vi "Path to String.vi"(1 "Path":path) -> (0 "Path String":string)   [LabVIEW 2020, in "feature_detection.lvlib" / "WeChat QR Code Detector.lvclass"]
uses:
  WeChat QR Code Detector.lvclass
  WeChat QR Code Detector.lvclass/WeChat QR Code Detector.ctl
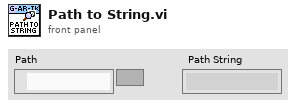
[diagram p1: front panel]
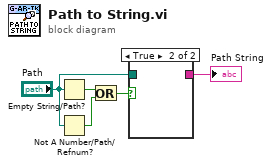
[diagram p0: block diagram]
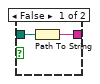
[diagram p2: hidden frame]
diagram:
  n1 = Empty String/Path?(string/path="Path") -> (empty?=w2:bool)
  n2 = Not A Number/Path/Refnum?(number/path/refnum="Path") -> (NaN/Path/Refnum?=w3:bool)
  n3 = Or(x=w2, y=w3) -> (x .or. y?=w1:bool)
  n4 = case shown="True" w1 {
    tunnel: [w7 _] -> w5
    tunnel: "Path" -> [w6 _]
    frame False {
      n5 = Path To String(path=w6) -> (string=w7:string)
    }
    frame True {
    }
  }
  "Path String" <- w5
